vi "Sine Wave PtByPt.vi"(1 "time":dbl format="%0.2f", 2 "phase":dbl format="%0.2f", 3 "frequency":dbl=1.0 format="%0.2f", 4 "amplitude":dbl=1.0 format="%0.2f") -> (0 "sine wave":dbl format="%0.2f")   [LabVIEW 2017, in "NI_PtbyPt.lvlib"]
doc: "Generates a sine wave point by point."
uses:
  <vilib>/ptbypt/NI_PtbyPt.lvlib
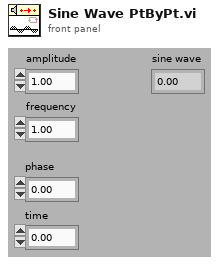
[diagram p1: front panel]
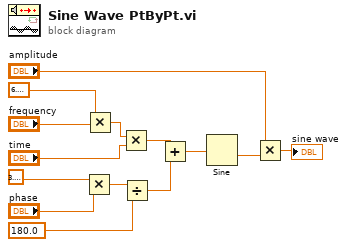
[diagram p0: block diagram]
diagram:
  n1 = Multiply(x=3.141592653589793, y="phase") -> (x*y=w9:dbl)
  n2 = Multiply(x=6.283185307179586, y="frequency") -> (x*y=w12:dbl)
  n3 = Multiply(x=w12, y="time") -> (x*y=w2:dbl)
  n4 = Divide(x=w9, y=180.0) -> (x/y=w1:dbl)
  n5 = Add(x=w2, y=w1) -> (x+y=w5:dbl)
  n6 = Sine(x=w5) -> (sin(x)=w4:dbl)
  n7 = Multiply(x="amplitude", y=w4) -> (x*y=→"sine wave":dbl)
